vi "XCtrl-State Changed.vi"(1 "Action":T1) -> (0 "Action 2":T1 caption="Action")   [LabVIEW 2010]
uses:
  <vilib>/_xctls/Action.ctl
  <vilib>/_xctls/XControlSupport.lvlib
panel:
  # "This is a handy utility VI I created for working with XControls. It isn't part of the XControl since I use it for several. It just encapsulates the setting of the State Changed boolean so I don't clutter up my block diagrams with a fairly large Bundle By Name node... I prefer Bundle by Name to Bundle in case the cluster gets modified in the future."
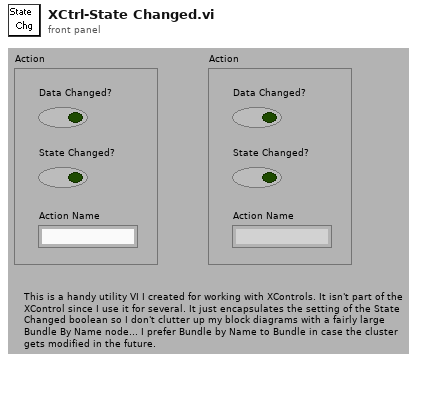
[diagram p1: front panel]
types:
  T1 = typedef "XControlSupport.lvlib/Action.ctl" = cluster{"Data Changed?":bool, "State Changed?":bool, "Action Name":string}
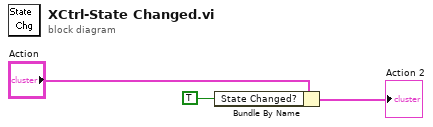
[diagram p0: block diagram]
diagram:
  n1 = Bundle By Name(cluster="Action", "State Changed?"=TRUE) -> (→"Action 2":T1)
